vi "Dequeue Controller Element.vi"(8 "error in (no error)":errorcluster, 11 "Message Queue":refnum<queue>) -> (0 "error out":errorcluster, 1 "Controller Queue Data":variant, 2 "Controller Queue Message":T1, 3 "dup Message Queue":refnum<queue>)   [LabVIEW 2017]
uses:
  Controller Queue Message Cluster.ctl
  Controller Queue Message.ctl
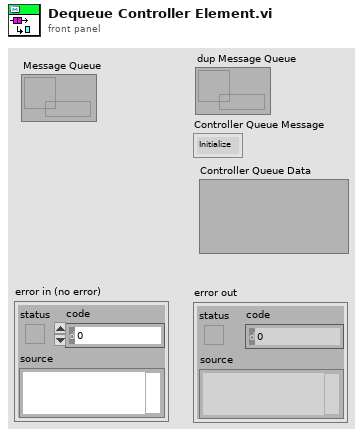
[diagram p1: front panel]
types:
  T1 = typedef "Controller Queue Message.ctl" = enum16{"Initialize", "Wait for First Request", "Start and Move", "Analysis", "Continue Travel", "Stop at Floor", "Open and Close Door Sequence", "No Request Remaining", "Emergency Call", "Terminate Process", "Error Handling"}
  T2 = typedef "Controller Queue Message Cluster.ctl" = cluster{"Controller Queue Message":T1, "Controller Queue Data":variant}
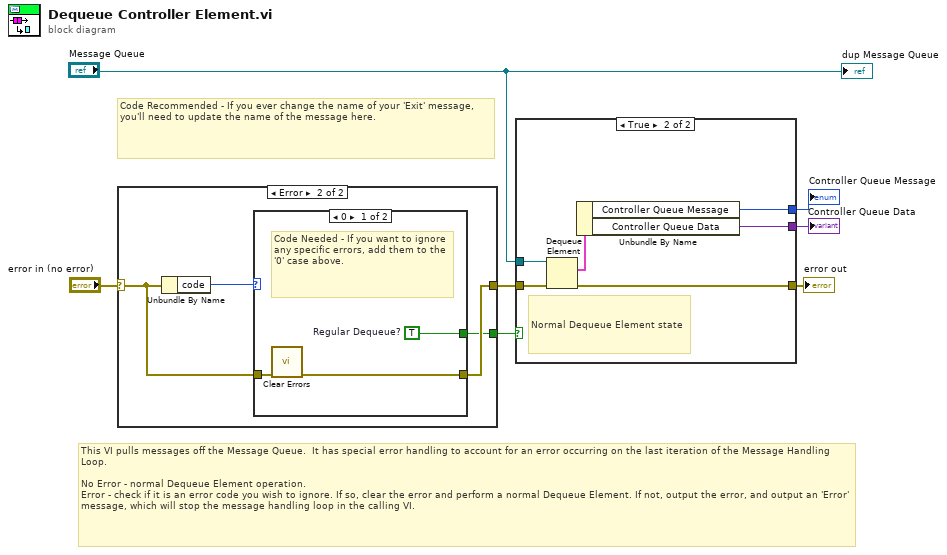
[diagram p0: block diagram]
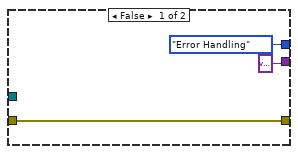
[diagram p2: hidden frame]
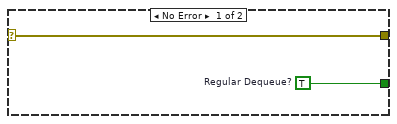
[diagram p3: hidden frame]
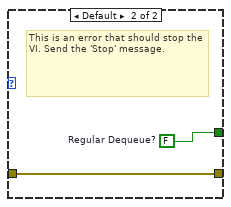
[diagram p4: hidden frame]
diagram:
  # "Code Recommended - If you ever change the name of your 'Exit' message, you'll need to update the name of the message here."
  # "This VI pulls messages off the Message Queue.  It has special error handling to account for an error occurring on the last iteration of the Message Handling Loop.\n\nNo Error - normal Dequeue Element operation.\nError - check if it is an error code you wish to ignore. If so, clear the error and perform a normal Dequeue Element. If not, output the error, and output an 'Error' message, which will stop the message handling loop in the calling VI."
  n1 = case shown="Error" "error in (no error)" {
    selector: "error in (no error)" -> [w9 w12]
    tunnel: [w9 w11] -> w5
    tunnel: [w8 w10] -> w4
    frame No Error {
      w8 = TRUE  # Regular Dequeue?
    }
    frame Error {
      n2 = Unbundle By Name(w12) -> ("code"=w13:i32)
      n3 = case shown="0" w13 {
        tunnel: [w16 w18] -> w11
        tunnel: w12 -> [w15 w18]
        tunnel: [w14 w17] -> w10
        frame 0 {
          w14 = TRUE  # Regular Dequeue?
          # "Code Needed - If you want to ignore any specific errors, add them to the '0' case above."
          n4 = call <vilib>:"Clear Errors.vi"("error in (no error)"=w15) -> ("error out"=w16:errorcluster)  [unwired: 5 in, 1 out]
        }
        frame Default {
          w17 = FALSE  # Regular Dequeue?
          # "This is an error that should stop the VI. Send the 'Stop' message."
        }
      }
    }
  }
  n5 = case shown="True" w4 {
    tunnel: [w21 w27] -> w6
    tunnel: w5 -> [w21 w26]
    tunnel: "Message Queue" -> [_ w24]
    tunnel: [variant ("Controller Queue Data") w23] -> w2
    tunnel: [Controller_Queue_Message."Error Handling" ("Controller Queue Message") w22] -> w1
    frame False {
    }
    frame True {
      # "Normal Dequeue Element state"
      n6 = Dequeue Element(queue=w24, error in (no error)=w26) -> (element=w25:T2, error out=w27:errorcluster)  [unwired: 1 in, 2 out]
      n7 = Unbundle By Name(w25) -> ("Controller Queue Message"=w22:T1, "Controller Queue Data"=w23:variant)
    }
  }
  "error out" <- w6
  "Controller Queue Data" <- w2
  "Controller Queue Message" <- w1
  "dup Message Queue" <- "Message Queue"
